vi "stage_get_travel_range.vi"(8 "error in (no error)":errorcluster, 11 "newport_xps in":refnum<class "newport_xps.lvclass">) -> (0 "error out":errorcluster, 1 "min(mm)":dbl, 2 "max (mm)":dbl, 3 "newport_xps out":refnum<class "newport_xps.lvclass">)   [LabVIEW 2015, in "newport_xps.lvclass"]
uses:
  newport_xps.lvclass
  newport_xps.lvclass/newport_xps.ctl
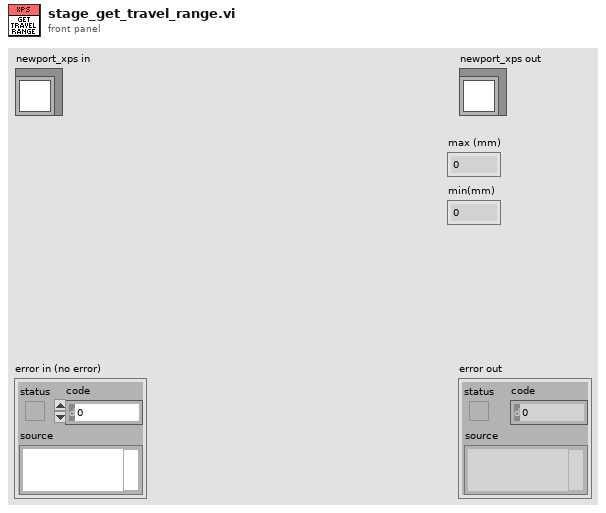
[diagram p1: front panel]
types:
  T1 = cluster{"connection TCP":refnum<k5>, "LogTo File":bool, "Log File refnum":refnum<file>, "no error if error log":bool}
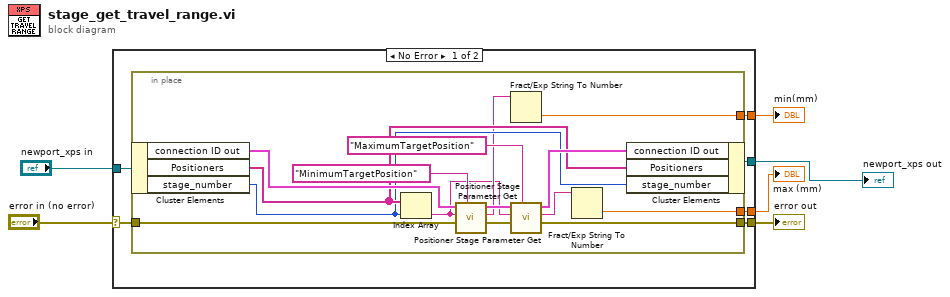
[diagram p0: block diagram]
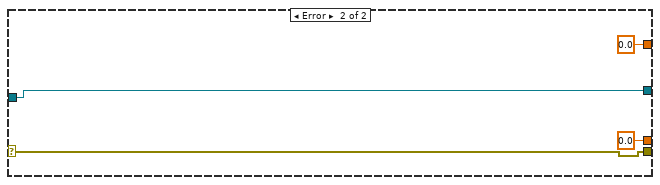
[diagram p2: hidden frame]
diagram:
  n1 = case shown="No Error" "error in (no error)" {
    selector: "error in (no error)" -> [w11 w29]
    tunnel: "newport_xps in" -> [w12 w28]
    tunnel: [w10 w29] -> w4
    tunnel: [w9 0.0] -> w3
    tunnel: [w8 0.0] -> w2
    tunnel: [w7 w28] -> w1
    frame No Error {
      n2 = in-place {
        in-place-border: w11 -> [w22]
        in-place-border: [w21] -> w10
        in-place-border: [w16] -> w9
        in-place-border: [w14] -> w8
        n3 = in-place-cluster #1(w12) -> ("connection ID out"=w26:T1, "Positioners"=w19:string[], "stage_number"=w18:i32)
        n4 = Index Array(array=w19, index=w18) -> (element=w13:string)
        n5 = call "Positioner Stage Parameter Get.vi"("Parameter Name (250 c max)"="MinimumTargetPosition", "XPS error in (no error)"=w22, "Positioner Name (250 c max)"=w13, "connection ID in"=w26) -> ("XPS error out"=w23:errorcluster, "Parameter Value"=w15:string, "connection ID out"=w25:T1)  [unwired: 4 in, 1 out]
        n6 = Fract/Exp String To Number(string=w15) -> (number=w14:dbl)  [unwired: 3 in, 1 out]
        n7 = call "Positioner Stage Parameter Get.vi"("Parameter Name (250 c max)"="MaximumTargetPosition", "XPS error in (no error)"=w23, "Positioner Name (250 c max)"=w13, "connection ID in"=w25) -> ("XPS error out"=w21:errorcluster, "Parameter Value"=w17:string, "connection ID out"=w20:T1)  [unwired: 4 in, 1 out]
        n8 = Fract/Exp String To Number(string=w17) -> (number=w16:dbl)  [unwired: 3 in, 1 out]
        n9 = in-place-cluster #1("connection ID out"=w20, "Positioners"=w19, "stage_number"=w18) -> (w7:refnum<class "newport_xps.lvclass">)
      }
    }
    frame Error {
    }
  }
  "error out" <- w4
  "newport_xps out" <- w1
  "min(mm)" <- w2
  "max (mm)" <- w3
